vi "Camera.v9.vi"() -> ()   [LabVIEW 2015]
uses:
  Camera Properties.ctl
  Microscope Settings.ctl
  CameraState.ctl
  ModeEnum.ctl
  Stack_State.ctl
  Stack Track.ctl
  CameraControlTypeDef.ctl
  <vilib>/DAQmx/write.llb/DAQmx Write (Digital 1D Wfm NChan NSamp).vi
  <vilib>/DAQmx/write.llb/DAQmx Write (Analog 1D Wfm NChan NSamp).vi
  <vilib>/DAQmx/create/channels.llb/DAQmx Create Channel (DO-Digital Output).vi
  <vilib>/DAQmx/create/channels.llb/DAQmx Create Channel (AO-Voltage-Basic).vi
  <vilib>/Waveform/WDTOps.llb/WDT Number of Waveform Samples DBL.vi
  <vilib>/DAQmx/configure/timing.llb/DAQmx Timing (Sample Clock).vi
  <vilib>/Waveform/DWDTOps.llb/DWDT Uncompress Digital.vi
  <vilib>/DAQmx/miscellaneous.llb/DAQmx Fill In Error Info.vi
  <vilib>/vision/NI_Vision_Development_Module.lvlib
panel:
  in  "Tab Control":enum32{"Camera Settings", "Recording"}(tab)
  in  "Microscope Settings Array":T1[](array[typedef]) {"Colour 2"."Filter" items=["Empty"=1, ""=2, ""=3, "561"=4, ""=5, "488"=6]; "Z Axis Stepping"."End" min=0.0 max=10.0 step=0.05; "Z Axis Stepping"."Step" min=0.0 max=10.0 step=0.05; "Z Axis Stepping"."Start" min=0.0 max=10.0 step=0.05; "ROI"."y" min=0.0 max=10.0 step=0.05; "ROI"."x" min=0.0 max=10.0 step=0.05; "ROI"."Width" min=0.0 max=10.0 step=0.05; "ROI"."Height" min=0.0 max=10.0 step=0.05; "Camera Delay" min=0.0 max=10.0 step=0.05; "Trigger Source" items=["Internal"=1.0, "External"=2.0]; "Readout Direction" items=["Internal"=1.0, "External"=2.0]; "Slit"."Scanning Mode" items=["Full Frame"=1.0, "Slit Scanning"=12.0]; "Piezo Position /um" min=0.0 max=10.0 step=0.05; "Relax/ms" min=0.0 max=10.0 step=0.05}
  in  "Scan":bool
  in  "Scan Continuously":bool
  out "error IO":errorcluster
  in  "Advanced DCAM Controls":i32(listbox) caption="Multicolumn Listbox"
  in  "Properties":T2=4211904 items=["SENSOR MODE"=4212128, "CCD MODE"=4212384, "READOUT MODE"=4211872, "ACTIVE VIEW INDEX"=4343136, "BITS PER CHANNEL"=4342976, "IMAGE PIXEL TYPE"=4343296, "BINNING"=4215968, "EXPOSURE TIME"=2049184, "CONTRAST GAIN"=3163312, "CONTRAST OFFSET"=3163328, "LIGHT MODE"=2114720, "SENSITIVITY"=2114992, "PHOTON IMAGING MODE"=2115200, "HIGH DYNAMIC RANGE MODE"=3163360, "WHITE BALANCE"=3163568, "TEMPERATURE"=2115232, "TEMPERATURE TARGET"=2115264, "SENSOR COOLER FAN"=2115296, "LINEBUNDLE HEIGHT"=4212192, "MECHANICAL SHUTTER"=2115488, "BACK FOCUS POSITION"=8422304, "TRIGGER CONNECTOR"=1066432, "TRIGGER SOURCE"=1066144, "OUTPUT TRIGGER SOURCE"=1852576, "TRIGGER GLOBAL EXPOSURE"=2049680, "FIRST TRIGGER BEHAVIOR"=2049696, "CHANNEL SYNC"=1852352, "READOUT DIRECTION"=4211904, "PRE HSYNC COUNT"=1852704, "INTERNAL LINE SPEED"=4191408, "INTERNAL LINE INVERVAL"=4191424]
  out "Image":T3(plugin-control)
  out "Histogram":T4(graph)
  in  "stop":bool
  in  "Signals Debugger":bool
  in  "Calibration":bool
  in  "MultiD Scan":bool
  in  "Stage Controller":bool
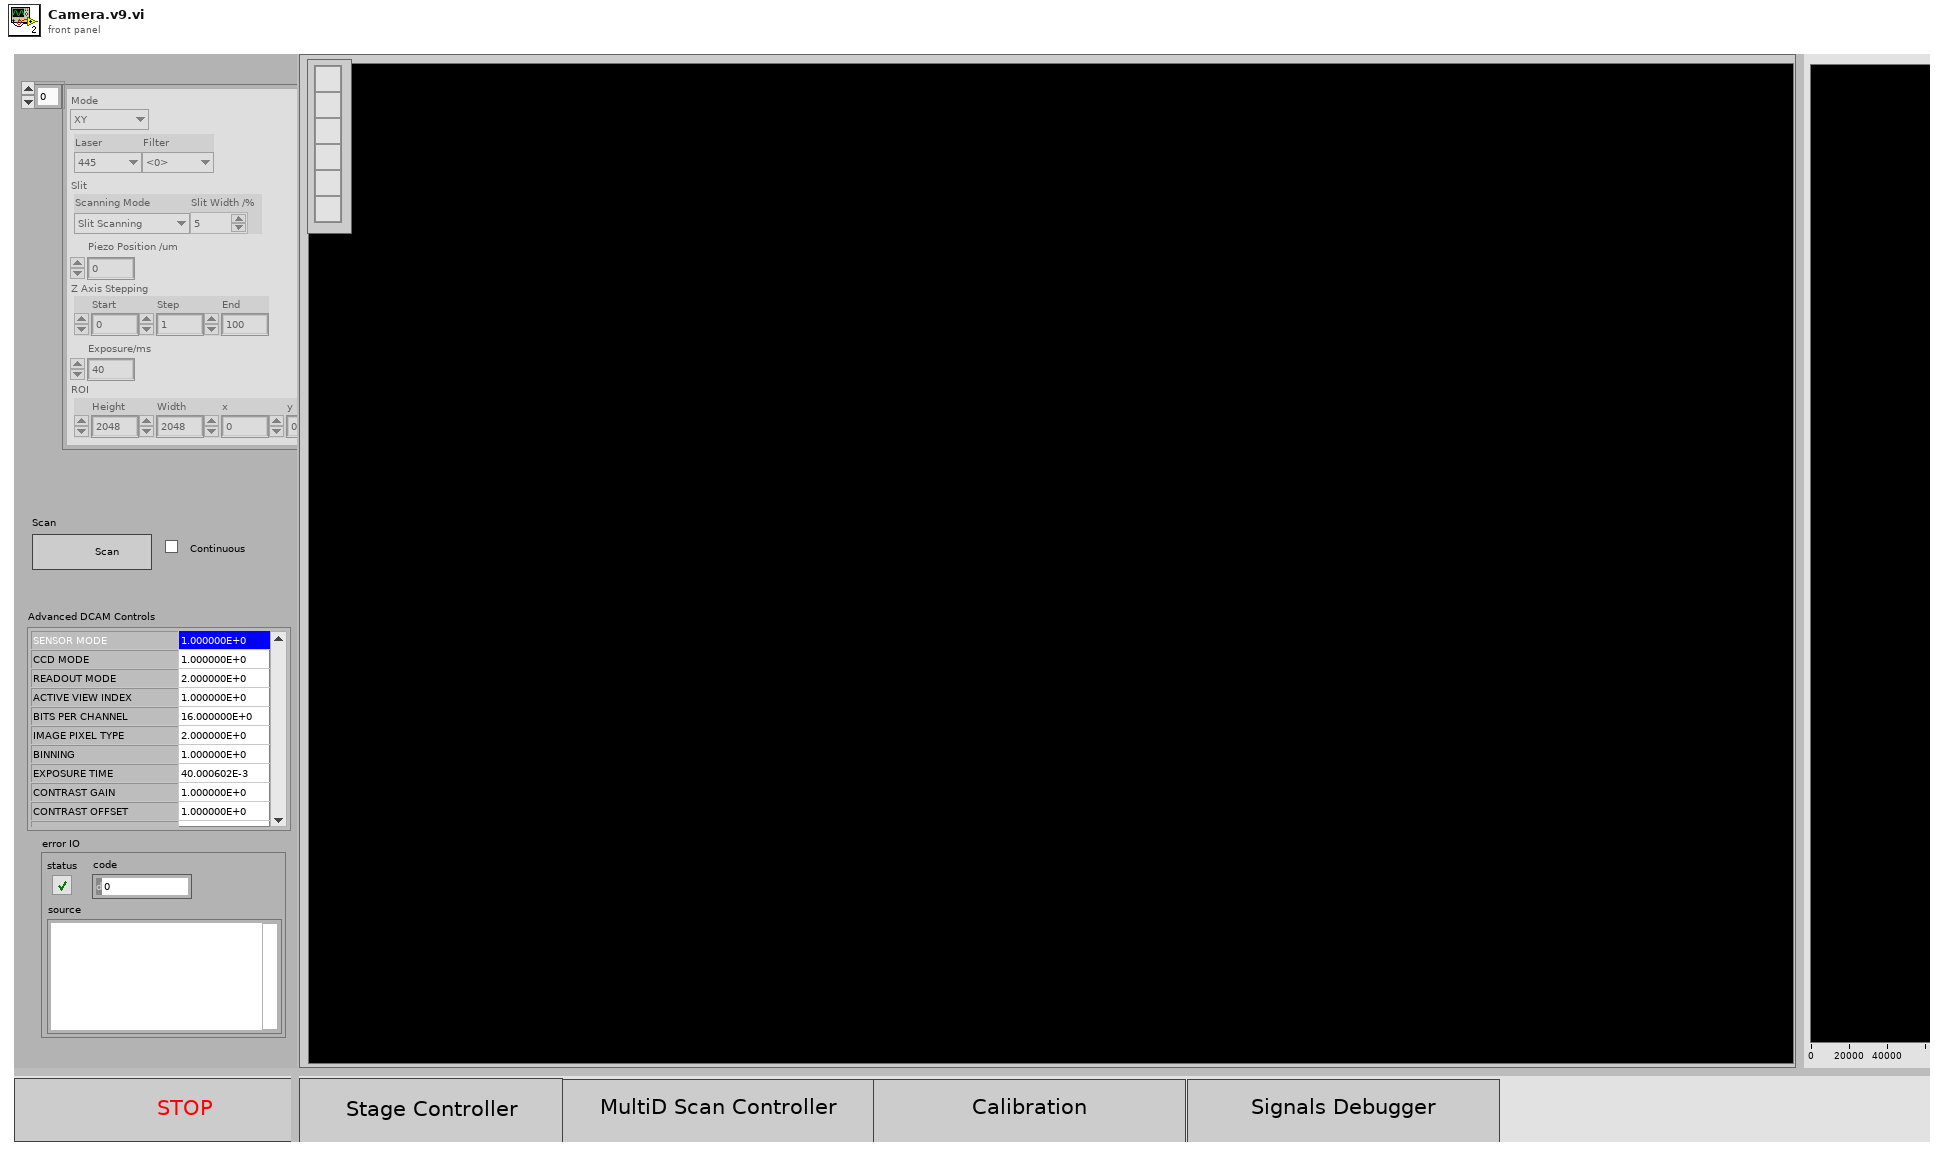
[diagram p1: front panel]
types:
  T1 = typedef "Microscope Settings.ctl" = cluster{"Mode":enum16{"X", "XY", "XYZ", "XYZT", "XYZC"}, "Colour 2":cluster{"Laser":enum16{"445", "488", "561", "647"}, "Filter":u16}, "Slit":cluster{"Scanning Mode":dbl, "Slit Width /%":dbl}, "Piezo Position /um":dbl, "Z Axis Stepping":cluster{"Start":dbl, "Step":dbl, "End":dbl}, "Exposure/ms":dbl, "ROI":cluster{"Height":dbl, "Width":dbl, "x":dbl, "y":dbl}, "Samples per millisecond":dbl, "Relax/ms":dbl, "Readout Direction":dbl, "Trigger Source":dbl, "Camera Delay":dbl}
  T2 = typedef "Camera Properties.ctl" = u32
  T3 = typedef "IMAQ Image.ctl" = refnum<image>
  T4 = cluster{"Starting Value":sgl, "Incremental Value":sgl, "Histogram":u32[]}
  T5 = cluster{"height":u32, "width":u32, "datatype":u32}
  T6 = typedef "CameraState.ctl" = enum16{"init", "active", "deinit"}
  T7 = typedef "ModeEnum.ctl" = enum16{"Idle", "generateWaves", "runWaves", "stop"}
  T8 = typedef "CameraControlTypeDef.ctl" = enum16{"Idle", "IntervalLineInt", "Ram Record", "HardDisk Record", "Disengage Update", "Update", "ROI", "Binning", "Scan Mode", "Trigger Mode", "Readout Mode", "Readout Direction", "Preview", "ROIWindow", "Trigger Source"}
  T9 = cluster{"Mode":u32, "Polarity":u32, "Times":u32, "Delay":dbl}
  T10 = typedef "Stack_State.ctl" = cluster{"State":T11, "Stack Number":i32, "Image":u16[][], "Stacks":i32}
  T11 = typedef "Stack Track.ctl" = enum16{"Idle", "Display", "Start Sequence", "Read Disk", "STOP", "Collecting", "End"}
  T12 = enum32{"Invalid", "Standard", "Closed", "Hidden", "Minimized", "Maximized"}
  T13 = typedef "Image Type" = u32
  T14 = cluster{"Enum":T8, "Microscope Settings Array":T1[]}
  T15 = cluster{"Mode":T7, "Microscope Settings Array":T1[]}
  T16 = cluster{"State":T11, "Timeout":i32, "Data 16":u16[][], "Timeout":i32}
  T17 = cluster{waveform(dbl)[], "Digital Waveform":digitalwaveform, "Digital Waveform":digitalwaveform}
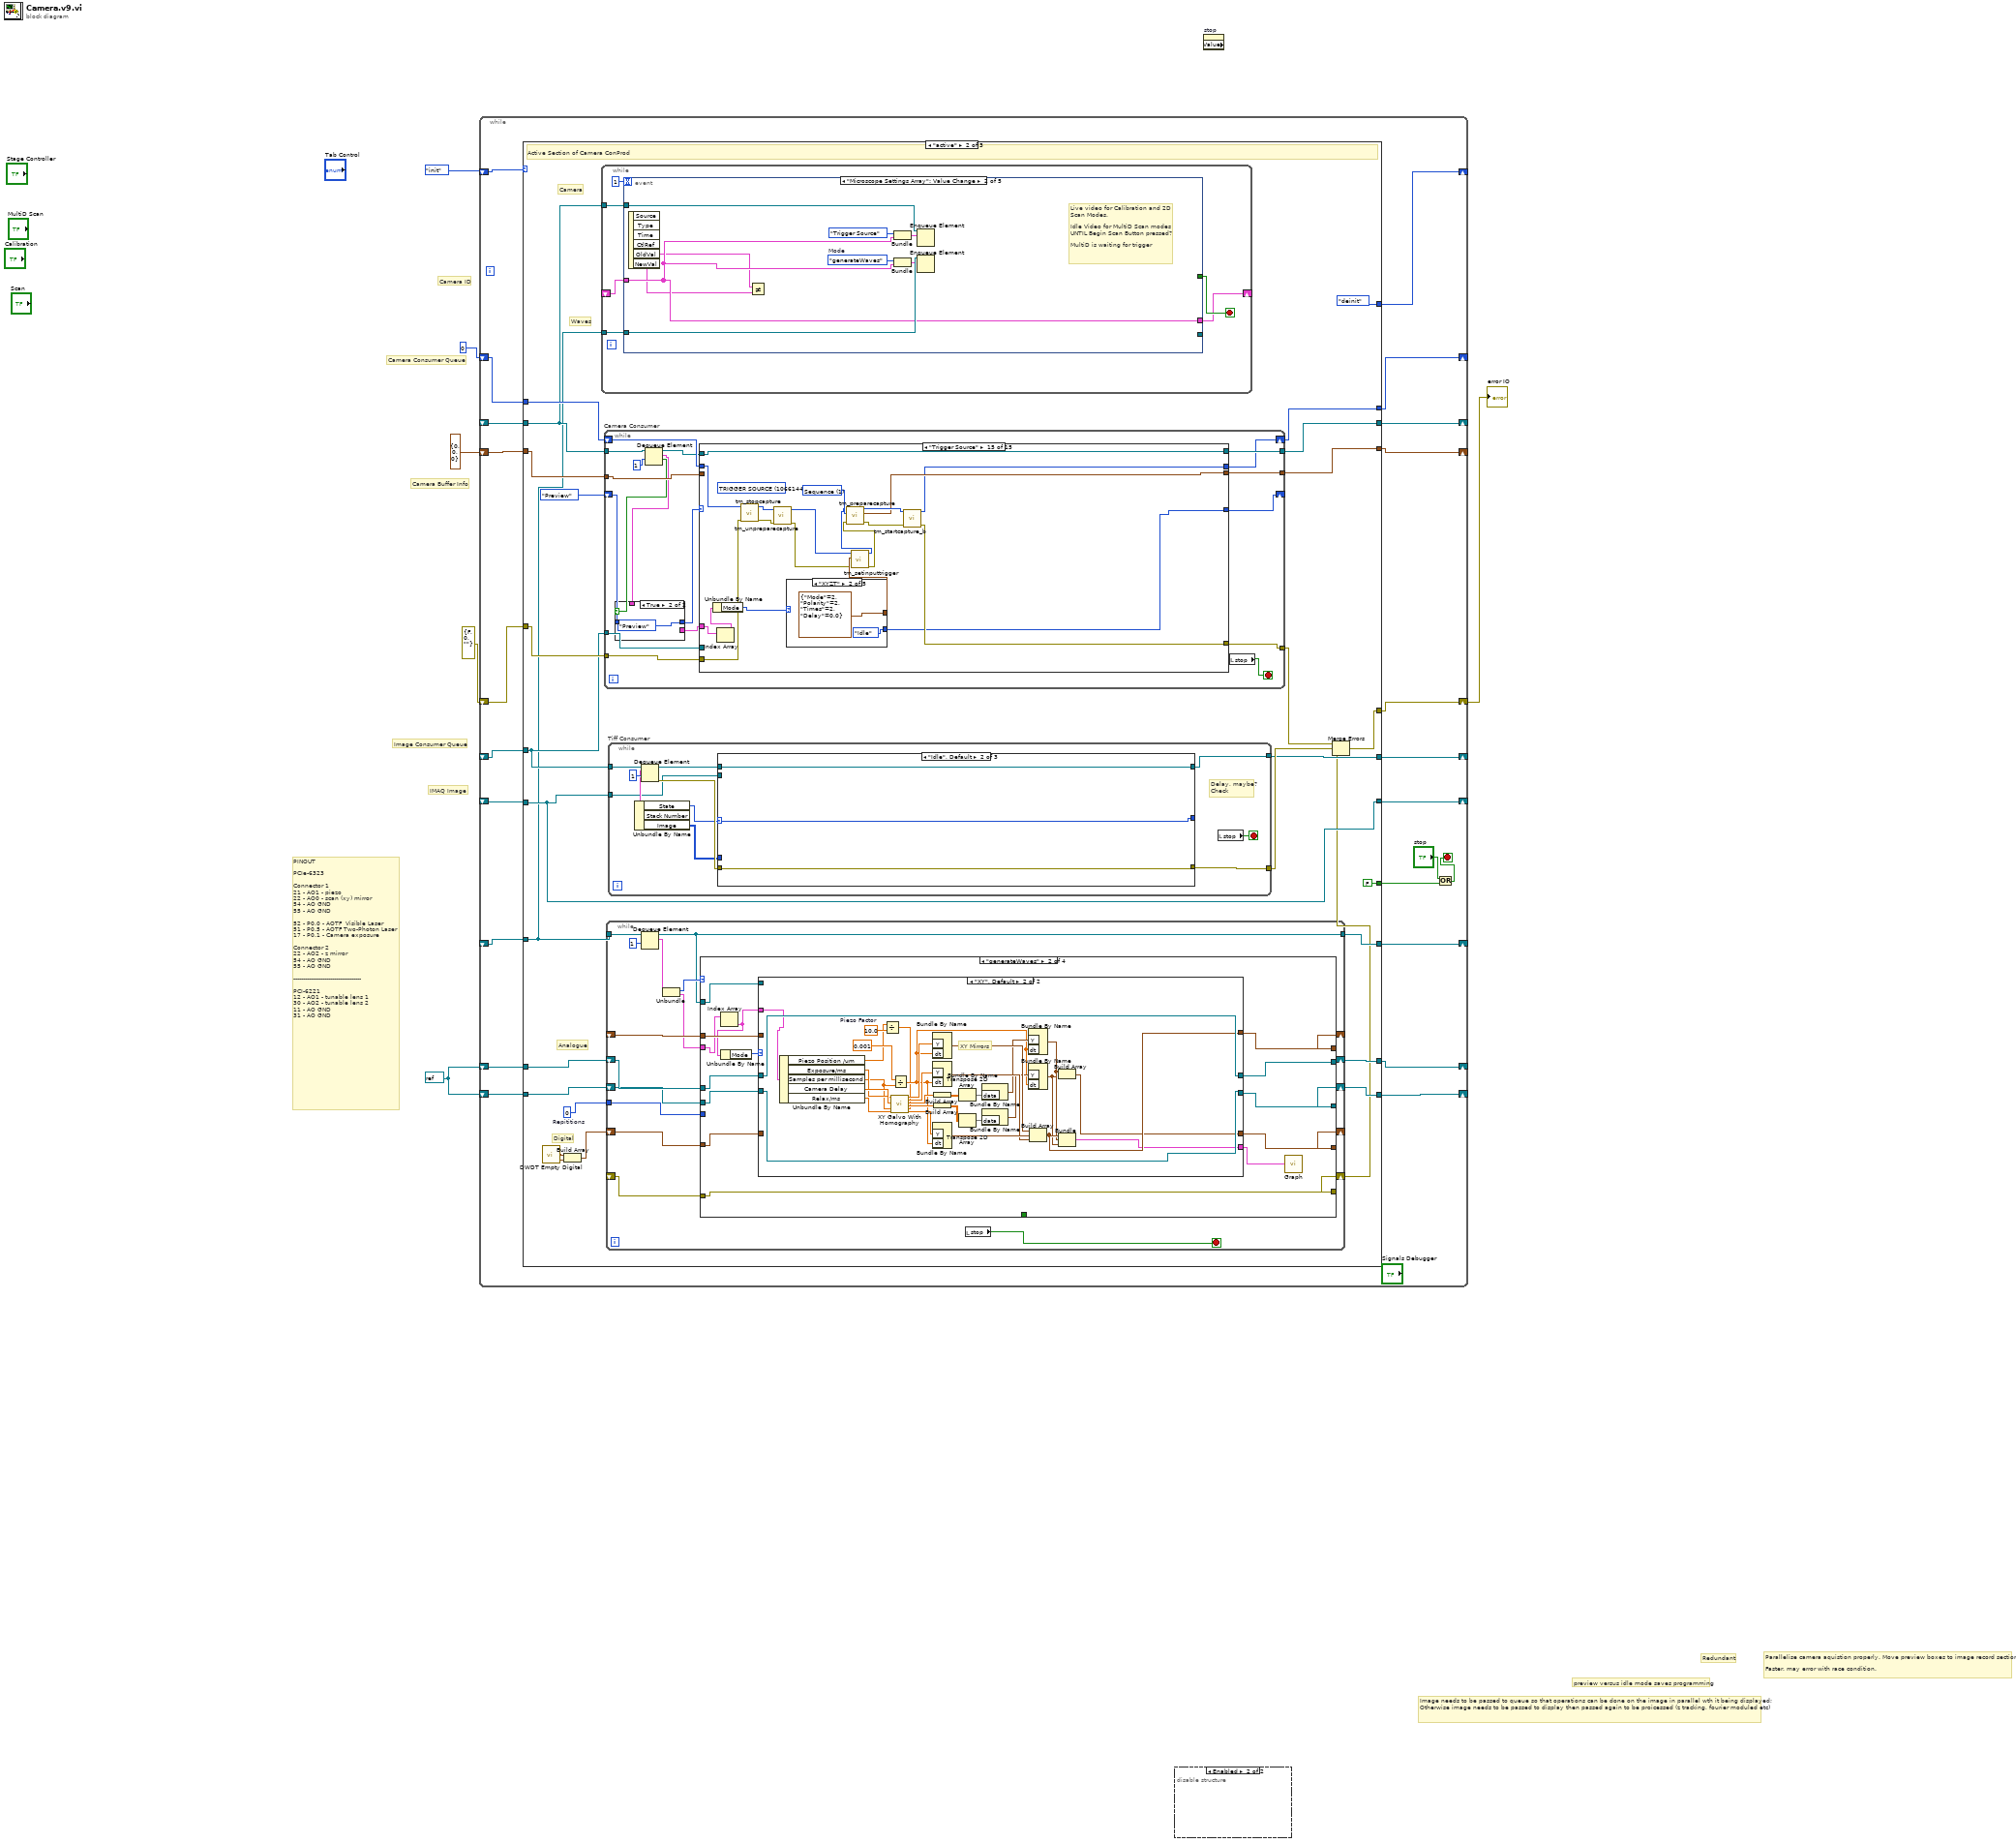
[diagram p0: block diagram]
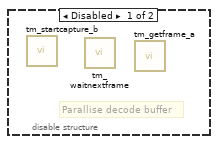
[diagram p2: hidden frame]
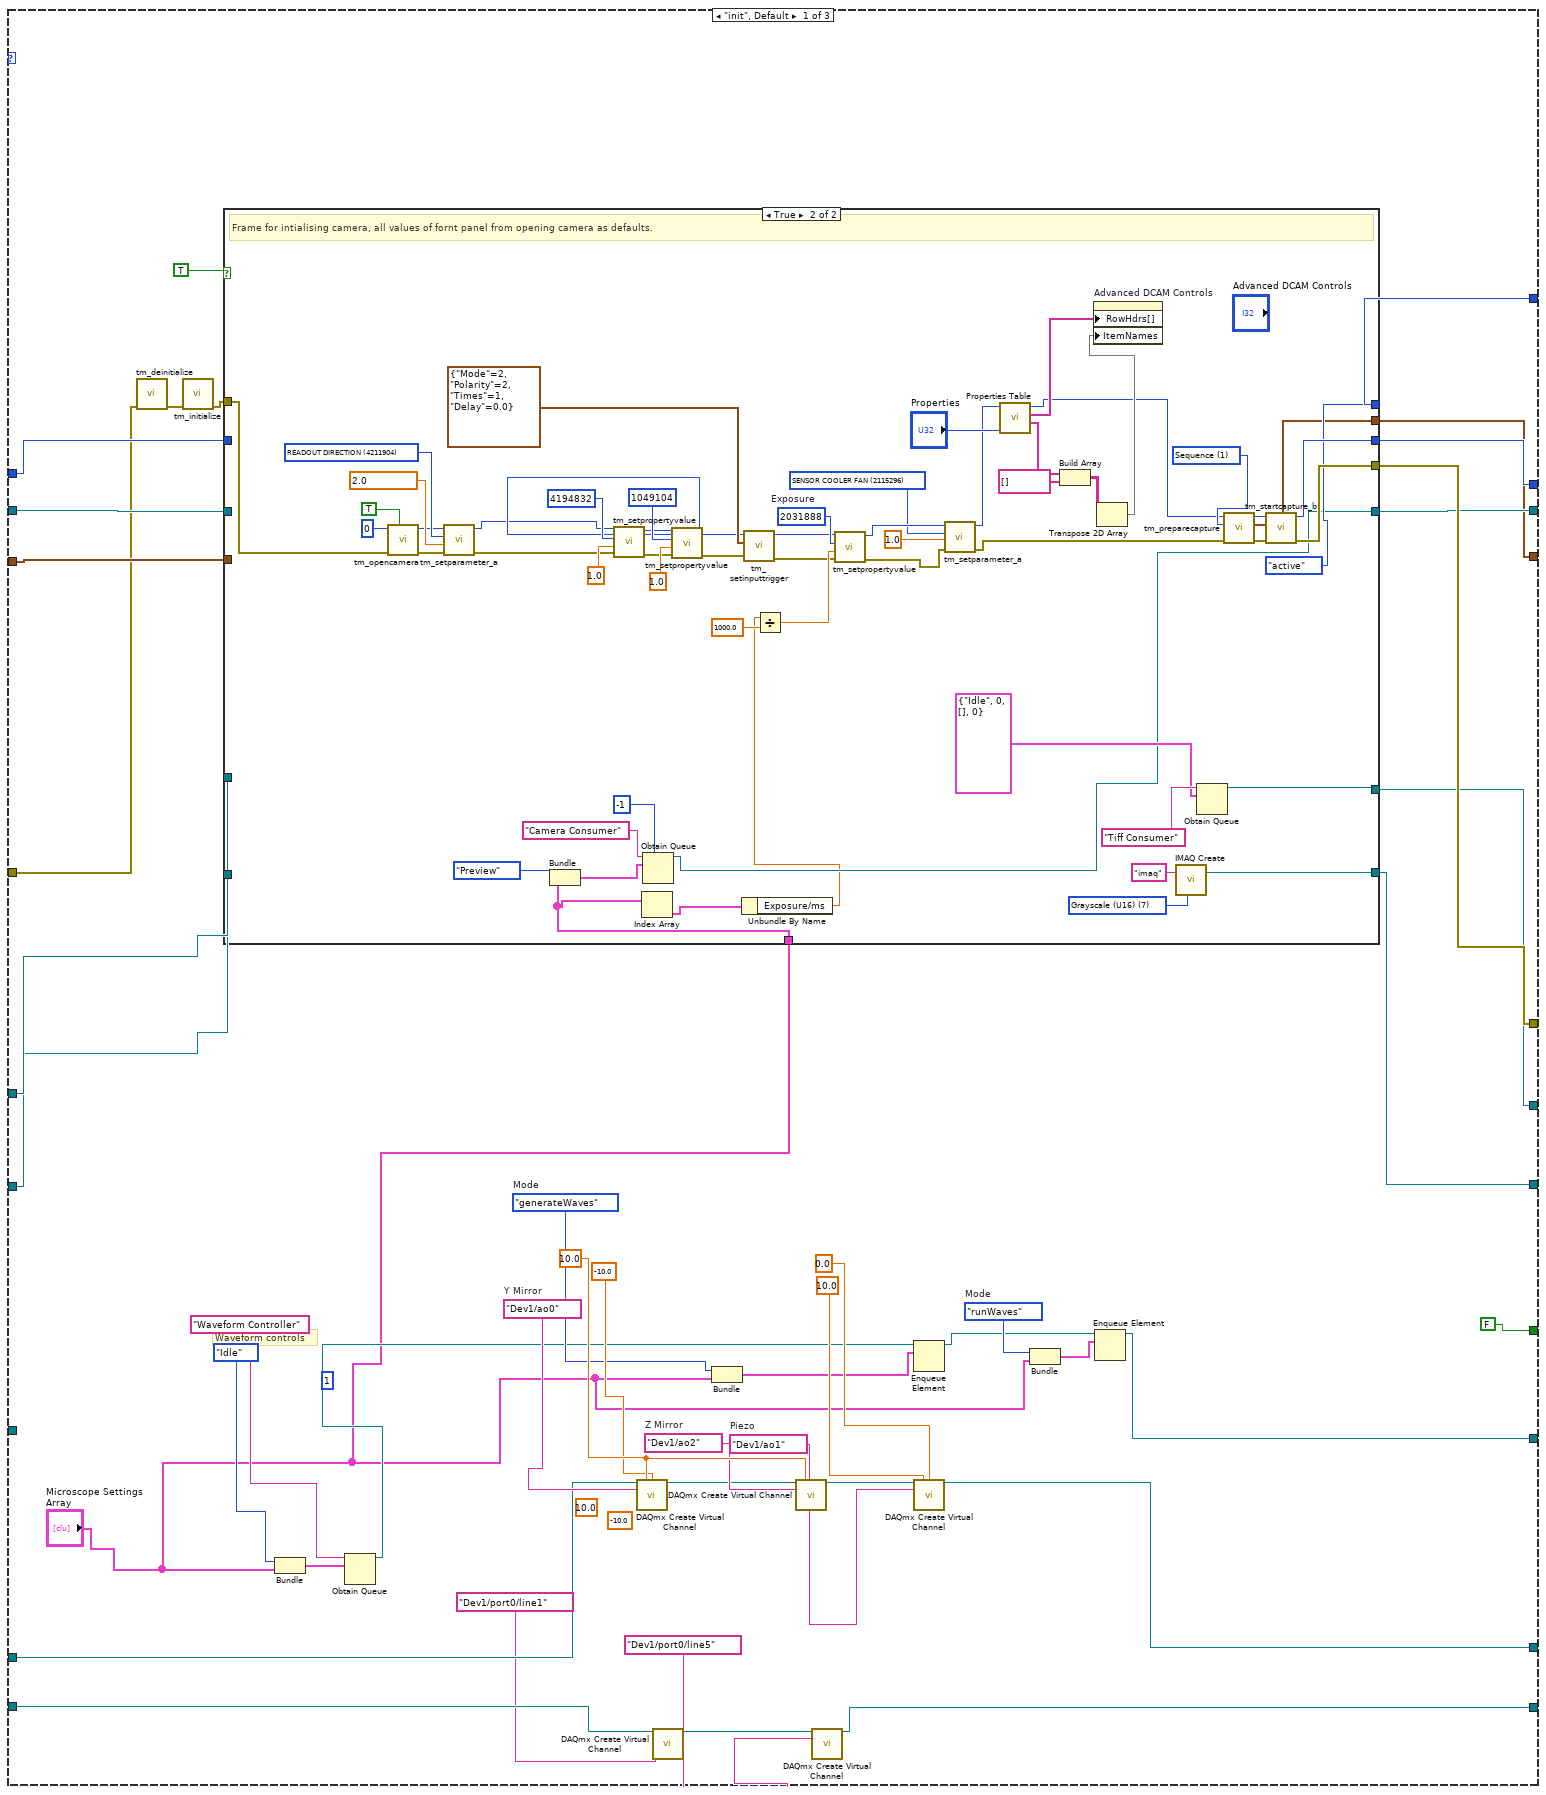
[diagram p3: hidden frame]
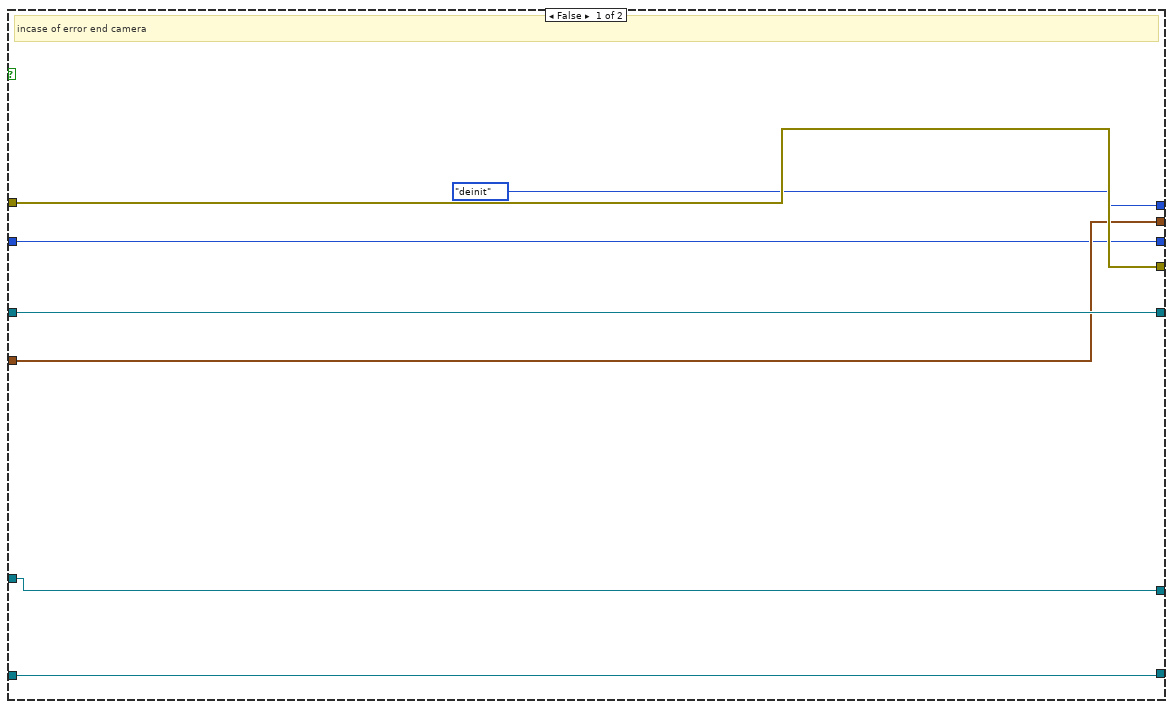
[diagram p4: hidden frame]
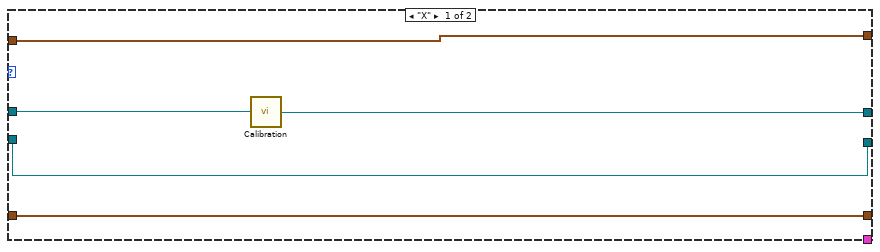
[diagram p6: hidden frame]
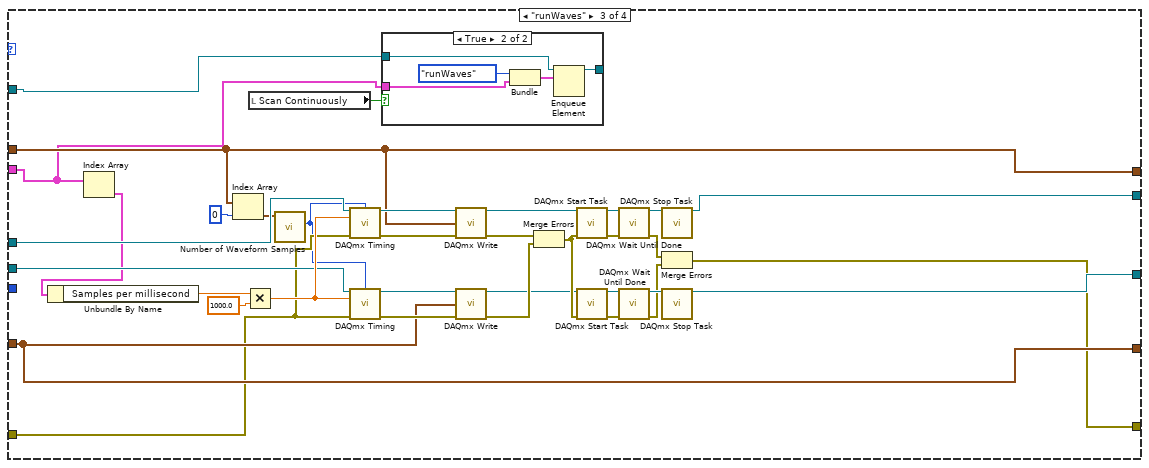
[diagram p7: hidden frame]
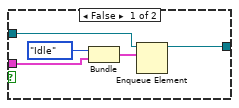
[diagram p8: hidden frame]
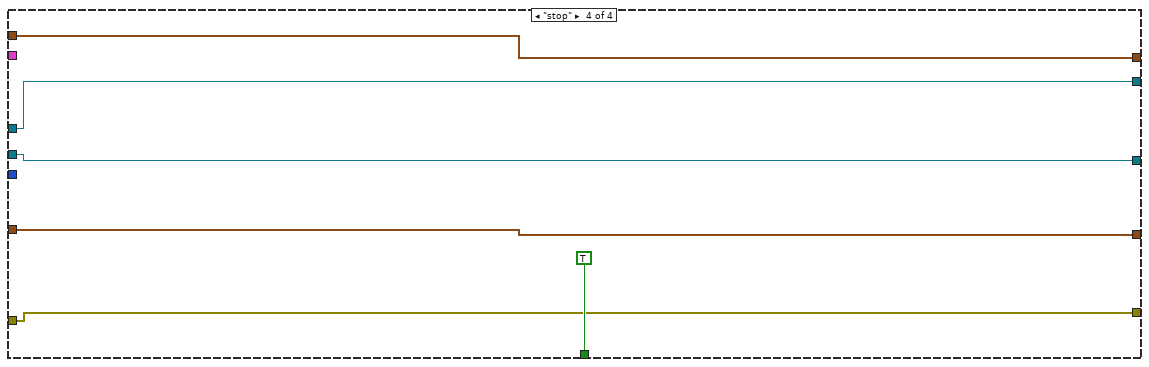
[diagram p9: hidden frame]
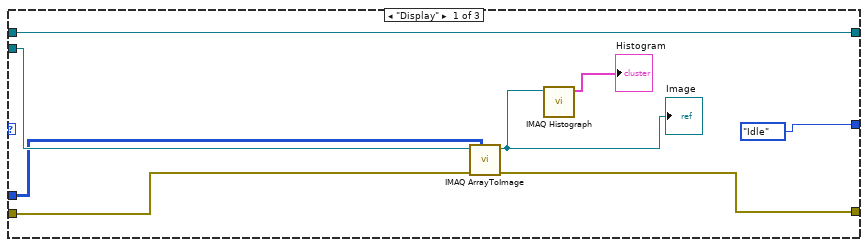
[diagram p10: hidden frame]
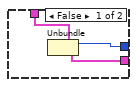
[diagram p12: hidden frame]
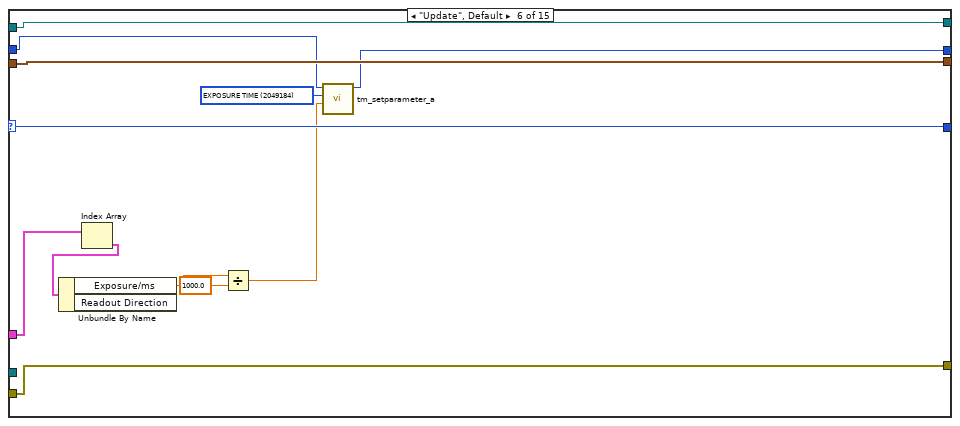
[diagram p18: hidden frame]
diagram:
  w3 = refnum<k21> refnum ("Mirror Z 2")
  # "PINOUT\n\nPCIe-6323\n\nConnector 1\n21 - AO1 - piezo\n22 - AO0 - scan (xy) mirror\n54 - AO GND\n55 - AO GND\n\n52 - P0.0 - AOTF  Visible Laser\n51 - P0.5 - AOTF Two-Photon Laser\n17 - P0.1 - Camera exposure\n\nConnector 2\n22 - AO2 - z mirror\n54 - AO GND\n55 - AO GND\n\n-----------------------------------\n\nPCI-6221\n12 - AO1 - tunable lens 1\n30 - AO2 - tunable lens 2\n11 - AO GND\n31 - AO GND"
  # "IMAQ Image"
  # "Camera Buffer Info"
  # "Image needs to be passed to queue so that operations can be done on the image in parallel wth it being displayed;\nOtherwise image needs to be passed to display then passed again to be proicessed (z tracking, fourier moduled etc)"
  # "preview versus idle mode saves programming"
  # "Parallelise camera aquistion properly. Move preview boxes to image record section.\n\nFaster. may error with race condition."
  # "Redundant"
  # "Image Consumer Queue"
  # "Camera Consumer Queue"
  # "Camera ID"
  n1 = while {
    shift-right: [w29] -> _
    shift-left: CameraState."init" -> [w28]
    shift-right: [w27] -> _
    shift-left: u32 0 ("Handle out") -> [w26]
    shift-right: [w25] -> w5
    shift-left: errorcluster {"status"=FALSE, "code"=0, "source"=""} ("error IO") -> [w24]
    shift-right: [w22] -> _
    shift-left: _ -> [w21]
    shift-right: [w23] -> _
    shift-left: _ -> [w20]
    shift-right: [w16] -> _
    shift-left: T5 {"height"=0, "width"=0, "datatype"=0} ("Buffer Info") -> [w15]
    shift-right: [w14] -> _
    shift-left: _ -> [w13]
    shift-right: [w12] -> _
    shift-left: w3 -> [w11]
    shift-right: [w9] -> _
    shift-left: w3 -> [w10]
    shift-right: [w8] -> _
    shift-left: _ -> [w7]
    stop <- w18 stop-if-true
    n2 = case shown="\"active\"" w28 {
      tunnel: [w71 CameraState."deinit" CameraState."init"] -> w29
      tunnel: [w70 w162 w555] -> w27
      tunnel: w26 -> [w48 w163 w555]
      tunnel: [w69 w161 w558] -> w25
      tunnel: w24 -> [w47 w155 w559]
      tunnel: [w68 w158 w542] -> w23
      tunnel: [w67 w157 w538] -> w22
      tunnel: w21 -> [w65 w150 w538]
      tunnel: w20 -> [w66 w148 w542]
      tunnel: [FALSE ("stop") FALSE ("stop") TRUE ("stop")] -> w17
      tunnel: [w63 w153 w552] -> w16
      tunnel: w15 -> [w62 w152 w552]
      tunnel: w13 -> [w60 w149 w551]
      tunnel: [w61 w149 w551] -> w14
      tunnel: w7 -> [_ w140 w537]
      tunnel: [w52 w141 w549] -> w12
      tunnel: w11 -> [w49 w144 w549]
      tunnel: w10 -> [w45 w143 w547]
      tunnel: [w40 w142 w547] -> w9
      tunnel: [w31 w139 w537] -> w8
      frame "init", Default {
        w35 = ModeEnum."runWaves"  # Mode
        (unwired) 1 ("max queue size (-1, unlimited)")
        w44 = ModeEnum."generateWaves"  # Mode
        (unwired) -10.0 ("minimum value")
        (unwired) 10.0 ("maximum value")
        w55 = tag "Dev1/ao1"  # Piezo
        w56 = tag "Dev1/ao2"  # Z Mirror
        w57 = tag "Dev1/ao0"  # Y Mirror
        w59 = 10.0 ("maximum value")
        # "Waveform controls"
        n3 = call "tm_deinitialize.vi"("error in (no error)"=w47) -> ("error out"=w73:errorcluster)  [unwired: 10 in]
        n4 = call "tm_initialize.vi"("error in (no error)"=w73) -> ("error out"=w72:errorcluster)  [unwired: 7 in, 3 out]
        n5 = case shown="True" TRUE {
          tunnel: w72 -> [w80 w102]
          tunnel: [CameraState."deinit" CameraState."active"] -> w71
          tunnel: [w80 w133] -> w69
          tunnel: [w75 w131] -> w70
          tunnel: [w78 w121] -> w68
          tunnel: [w77 w128] -> w67
          tunnel: w66 -> [w78 _]
          tunnel: w65 -> [w77 _]
          tunnel: [w76 w126] -> w63
          tunnel: w62 -> [w76 _]
          tunnel: w48 -> [w75 _]
          tunnel: [w74 w123] -> w61
          tunnel: w60 -> [w74 _]
          tunnel: "Microscope Settings Array" -> [_ w81]
          frame False {
            # "incase of error end camera"
          }
          frame True {
            w99 = u32 2115296 items=["SENSOR MODE"=4212128, "CCD MODE"=4212384, "READOUT MODE"=4211872, "ACTIVE VIEW INDEX"=4343136, "BITS PER CHANNEL"=4342976, "IMAGE PIXEL TYPE"=4343296, "BINNING"=4215968, "EXPOSURE TIME"=2049184, "CONTRAST GAIN"=3163312, "CONTRAST OFFSET"=3163328, "LIGHT MODE"=2114720, "SENSITIVITY"=2114992, "PHOTON IMAGING MODE"=2115200, "HIGH DYNAMIC RANGE MODE"=3163360, "WHITE BALANCE"=3163568, "TEMPERATURE"=2115232, "TEMPERATURE TARGET"=2115264, "SENSOR COOLER FAN"=2115296, "LINEBUNDLE HEIGHT"=4212192, "MECHANICAL SHUTTER"=2115488, "BACK FOCUS POSITION"=8422304, "TRIGGER CONNECTOR"=1066432, "TRIGGER SOURCE"=1066144, "OUTPUT TRIGGER SOURCE"=1852576, "TRIGGER GLOBAL EXPOSURE"=2049680, "FIRST TRIGGER BEHAVIOR"=2049696, "CHANNEL SYNC"=1852352, "READOUT DIRECTION"=4211904, "PRE HSYNC COUNT"=1852704, "INTERNAL LINE SPEED"=4226000, "INTERNAL LINE INTERVAL"=4226016] ("Parameter")
            w108 = u32 2031888  # Exposure
            w119 = sgl 2.0 items=["Forward"=1.0, "Backward"=2.0] ("Readout Direction")
            w120 = u32 4211904 items=["SENSOR MODE"=4212128, "CCD MODE"=4212384, "READOUT MODE"=4211872, "ACTIVE VIEW INDEX"=4343136, "BITS PER CHANNEL"=4342976, "IMAGE PIXEL TYPE"=4343296, "BINNING"=4215968, "EXPOSURE TIME"=2049184, "CONTRAST GAIN"=3163312, "CONTRAST OFFSET"=3163328, "LIGHT MODE"=2114720, "SENSITIVITY"=2114992, "PHOTON IMAGING MODE"=2115200, "HIGH DYNAMIC RANGE MODE"=3163360, "WHITE BALANCE"=3163568, "TEMPERATURE"=2115232, "TEMPERATURE TARGET"=2115264, "SENSOR COOLER FAN"=2115296, "LINEBUNDLE HEIGHT"=4212192, "MECHANICAL SHUTTER"=2115488, "BACK FOCUS POSITION"=8422304, "TRIGGER CONNECTOR"=1066432, "TRIGGER SOURCE"=1066144, "OUTPUT TRIGGER SOURCE"=1852576, "TRIGGER GLOBAL EXPOSURE"=2049680, "FIRST TRIGGER BEHAVIOR"=2049696, "CHANNEL SYNC"=1852352, "READOUT DIRECTION"=4211904, "PRE HSYNC COUNT"=1852704, "INTERNAL LINE SPEED"=4226000, "INTERNAL LINE INTERVAL"=4226016] ("Parameter")
            w125 = T13 7 items=["Grayscale (U8)", "Grayscale (I16)", "Grayscale (SGL)", "Complex (CSG)", "RGB (U32)", "HSL (U32)", "RGB (U64)", "Grayscale (U16)"] ("Image Type")
            w135 = 1 items=["Snap", "Sequence"] ("Capture mode")
            # "Frame for intialising camera, all values of fornt panel from opening camera as defaults."
            n6 = call "tm_opencamera.vi"("Force Open"=TRUE, "error in (no error)"=w102, "Camera Index"=u32 0) -> ("error out"=w117:errorcluster, "Handle out"=w118:u32)  [unwired: 6 in, 1 out]
            n7 = call "tm_setparameter_a.vi"("error in (no error)"=w117, "Value in"=w119, "Parameter"=w120, "Handle in"=w118) -> ("error out"=w88:errorcluster, "Handle out"=w109:u32)  [unwired: 6 in]
            n8 = Bundle("Enum"=CameraControlTypeDef."Preview", "Microscope Settings Array"=w81) -> (w103:T14)  [unwired: 1 in]
            n9 = call "tm_setpropertyvalue.vi"("error in (no error)"=w88, "Value in"=sgl 1.0, "Property ID"=u32 4194832, "Handle in"=w109) -> ("error out"=w87:errorcluster, "Handle out"=w112:u32)  [unwired: 6 in]
            n10 = Index Array(array=w81) -> (element=w82:T1)  [unwired: 1 in]
            n11 = Obtain Queue(max queue size (-1, unlimited)=-1, name (unnamed)="Camera Consumer", element data type=w103) -> (queue out=w121:refnum<queue>)  [unwired: 2 in, 2 out]
            n12 = call "tm_setpropertyvalue.vi"("error in (no error)"=w87, "Value in"=sgl 1.0, "Property ID"=u32 1049104, "Handle in"=w112) -> ("error out"=w86:errorcluster, "Handle out"=w110:u32)  [unwired: 6 in]
            n13 = Unbundle By Name(w82) -> ("Exposure/ms"=w89:dbl)
            n14 = call <userlib>:"tm_setinputtrigger.vi"("error in (no error)"=w86, "Parameters"=T9 {"Mode"=2, "Polarity"=2, "Times"=1, "Delay"=0.0}, "Handle in"=w110) -> ("error out"=w85:errorcluster, "Handle out"=w107:u32)  [unwired: 7 in]
            n15 = Divide(x=w89, y=sgl 1000.0) -> (x/y=w105:dbl)
            n16 = call "tm_setpropertyvalue.vi"("error in (no error)"=w85, "Value in"=w105, "Property ID"=w108, "Handle in"=w107) -> ("error out"=w84:errorcluster, "Handle out"=w100:u32)  [unwired: 6 in]
            n17 = call "tm_setparameter_a.vi"("error in (no error)"=w84, "Value in"=1.0, "Parameter"=w99, "Handle in"=w100) -> ("error out"=w83:errorcluster, "Handle out"=w91:u32)  [unwired: 6 in]
            n18 = call "Properties Table.vi"("Properties"="Properties", "Handle In"=w91) -> ("Value Stirngs Out"=w95:string[], "Row Headers"=w96:string[], "Handle Out"=w90:u32)  [unwired: 3 in, 1 out]
            n19 = Build Array(w95, string[] [] ("element")) -> (w93:string[][])
            n20 = Transpose 2D Array(2D array=w93) -> (transposed array=w92:string[][])
            n21 = property on="Advanced DCAM Controls" class="MCListbox (strict)"("RowHdrs[]"=w96, "ItemNames"=w92) -> ()  [unwired: 2 in, 2 out]
            n22 = call "IMAQ Create"("Image Name"="imaq", "Image Type"=w125) -> ("New Image"=w123:T3)  [unwired: 3 in, 1 out]
            n23 = Obtain Queue(name (unnamed)="Tiff Consumer", element data type=T10 {"State"=enum."Idle", "Stack Number"=0, "Image"=[], "Stacks"=0} ("input cluster")) -> (queue out=w128:refnum<queue>)  [unwired: 3 in, 2 out]
            n24 = call "tm_preparecapture.vi"("error in (no error)"=w83, "Capture mode"=w135, "Handle in"=w90) -> ("error out"=w134:errorcluster, "Buffer Info"=w126:T5, "Handle out"=w132:u32)  [unwired: 5 in, 1 out]
            n25 = call "tm_startcapture_b.vi"("error in (no error)"=w134, "Handle in"=w132) -> ("error out"=w133:errorcluster, "Handle out"=w131:u32)  [unwired: 8 in]
          }
        }
        n26 = Bundle("Mode"=ModeEnum."Idle", "Microscope Settings Array"="Microscope Settings Array") -> (w42:T15)  [unwired: 1 in]
        n27 = Obtain Queue(name (unnamed)="Waveform Controller", element data type=w42) -> (queue out=w41:refnum<queue>)  [unwired: 3 in, 2 out]
        n28 = call-poly <vilib>:"DAQmx Create Virtual Channel.vi"("task in"=w49, "maximum value"=w59, "minimum value"=-10.0, "physical channels"=w57) -> ("task out"=w51:refnum<k21>)  [unwired: 10 in, 1 out]
        n29 = call-poly <vilib>:"DAQmx Create Virtual Channel.vi"("task in"=w45, "lines"=tag "Dev1/port0/line1") -> ("task out"=w46:refnum<k21>)  [unwired: 12 in, 1 out]
        n30 = Bundle("Mode"=w44, "Microscope Settings Array"="Microscope Settings Array") -> (w33:T15)  [unwired: 1 in]
        n31 = call-poly <vilib>:"DAQmx Create Virtual Channel.vi"("task in"=w51, "maximum value"=w59, "physical channels"=w56) -> ("task out"=w50:refnum<k21>)  [unwired: 11 in, 1 out]
        n32 = call-poly <vilib>:"DAQmx Create Virtual Channel.vi"("task in"=w46, "lines"=tag "Dev1/port0/line5") -> ("task out"=w40:refnum<k21>)  [unwired: 12 in, 1 out]
        n33 = Enqueue Element(queue=w41, element=w33) -> (queue out=w34:refnum<queue>)  [unwired: 2 in, 2 out]
        n34 = call-poly <vilib>:"DAQmx Create Virtual Channel.vi"("task in"=w50, "maximum value"=10.0 ("minimum value"), "minimum value"=0.0 ("maximum value"), "physical channels"=w55) -> ("task out"=w52:refnum<k21>)  [unwired: 10 in, 1 out]
        n35 = Bundle("Mode"=w35, "Microscope Settings Array"="Microscope Settings Array") -> (w32:T15)  [unwired: 1 in]
        n36 = Enqueue Element(queue=w34, element=w32) -> (queue out=w31:refnum<queue>)  [unwired: 2 in, 2 out]
      }
      frame "active" {
        w147 = 0  # Repititions
        # "Waves"
        # "Camera"
        # "Digital"
        # "Analogue"
        # "Active Section of Camera ConProd"
        n37 = call <vilib>:"DWDT Empty Digital.vi"() -> ("digital waveform out"=w145:digitalwaveform)  [unwired: 5 in]
        n38 = Build Array(w145, w145) -> (w146:digitalwaveform[])
        n39 = while {
          tunnel: w148 -> [w503]
          shift-right: [w502] -> _
          shift-left: _ -> [w501]
          tunnel: w140 -> [w499]
          stop <- w504 stop-if-true
          n40 = event shown="[1] \"Microscope Settings Array\": Value Change" {
            selector: _ -> [_ _ _ _ _]
            dyn-events: _ -> [_ _ _ _ _]
            timeout: 1 -> [_ _ _ _ _]
            tunnel: [w512 _ _ _ _] -> w504
            tunnel: w503 -> [w507 w521 _ _ _]
            tunnel: [w505 w515 _ _ w536] -> w502
            tunnel: w501 -> [w505 w515 _ w529 _]
            tunnel: [_ _ _ w528 _] -> _
            tunnel: w499 -> [w506 w520 _ w527 _]
            event "stop": Value Change {
              w510 = ModeEnum."stop"  # Mode
              n41 = event-data() -> ()  [unwired: 1 in, 6 out]
              n42 = Bundle("Enum"=CameraControlTypeDef."Idle", "Value"=w505) -> (w508:cluster{"Enum":T8, "Value":T1[]})  [unwired: 1 in]
              n43 = Bundle("Mode"=w510, "Value"=w505) -> (w509:cluster{"Mode":T7, "Value":T1[]})  [unwired: 1 in]
              n44 = Enqueue Element(queue=w507, element=w508) -> ()  [unwired: 2 in, 3 out]
              n45 = Enqueue Element(queue=w506, element=w509) -> ()  [unwired: 2 in, 3 out]
              n46 = local read "stop"() -> (w512:bool)
            }
            event "Microscope Settings Array": Value Change {
              w518 = ModeEnum."generateWaves"  # Mode
              # "Live video for Calibration and 2D\nScan Modes.\n\nIdle Video for MultiD Scan modes\nUNTIL Begin Scan Button pressed?\n\nMultiD is waiting for trigger"
              n47 = event-data() -> ("OldVal"=w514:T1[], "NewVal"=w513:T1[])  [unwired: 1 in, 4 out]
              n48 = Not Equal?(x=w514, y=w513) -> ()  [unwired: 1 out]
              n49 = Bundle("Enum"=CameraControlTypeDef."Trigger Source", "Value"=w515) -> (w516:cluster{"Enum":T8, "Value":T1[]})  [unwired: 1 in]
              n50 = Bundle("Mode"=w518, "Value"=w515) -> (w517:cluster{"Mode":T7, "Value":T1[]})  [unwired: 1 in]
              n51 = Enqueue Element(queue=w521, element=w516) -> ()  [unwired: 2 in, 3 out]
              n52 = Enqueue Element(queue=w520, element=w517) -> ()  [unwired: 2 in, 3 out]
            }
            event "Signals Debugger": Value Change {
              n53 = event-data() -> ()  [unwired: 1 in, 6 out]
              n54 = disable-structure shown="Disabled" {
                frame Disabled {
                  n55 = control-ref of="stop"() -> (w525:refnum<vi>)
                  n56 = call "PopOutGraph.vi"("OK Button 2"=w525) -> ()  [unwired: 2 in]
                }
                frame Enabled {
                }
              }
              n57 = vi-ref "Graph.vi"() -> (w522:refnum<vi>)
              n58 = invoke class="VI" method="FP.Open"(reference=w522, "Activate"=TRUE ("Front Panel Window:Open"), "State"=T12."Standard") -> ()  [unwired: 2 in, 5 out]
            }
            event "Scan": Value Change {
              n59 = event-data() -> ("NewVal"=w526:bool)  [unwired: 1 in, 5 out]
              n60 = case shown="True" w526 {
                tunnel: w529 -> [_ w535]
                tunnel: [w530 w534] -> w528
                tunnel: w527 -> [w530 w533]
                frame False {
                }
                frame True {
                  w532 = ModeEnum."runWaves"  # Mode
                  n61 = Bundle("Mode"=w532, "Value"=w535) -> (w531:cluster{"Mode":T7, "Value":T1[]})  [unwired: 1 in]
                  n62 = Enqueue Element(queue=w533, element=w531) -> (queue out=w534:refnum<queue>)  [unwired: 2 in, 2 out]
                }
              }
            }
            event Timeout {
              n63 = event-data() -> ()  [unwired: 1 in, 3 out]
              n64 = property on="Microscope Settings Array" class="Arr (strict)"() -> ("Value"=w536:T1[])  [unwired: 2 in, 2 out]
            }
          }
        }
        n65 = while "Camera Consumer" {
          tunnel: w155 -> [w329]
          tunnel: [w314] -> w159
          tunnel: w148 -> [w322]
          tunnel: [w330] -> w158
          shift-right: [w328] -> _
          shift-left: CameraControlTypeDef."Preview" ("Enum") -> [w318]
          tunnel: [w325] -> w153
          tunnel: w152 -> [w324]
          tunnel: w150 -> [w317]
          shift-right: [w326] -> w162
          shift-left: w163 -> [w327]
          stop <- w313 stop-if-true
          n66 = Dequeue Element(queue=w322, timeout in ms (-1)=1) -> (queue out=w321:refnum<queue>, element=w316:T14, timed out?=w320:bool)  [unwired: 1 in, 1 out]
          n67 = case shown="True" w320 {
            tunnel: [w332 CameraControlTypeDef."Preview" ("Enum")] -> w319
            tunnel: w318 -> [_ _]
            tunnel: w316 -> [w333 _]
            tunnel: [w331 _] -> w315
            frame False {
              n68 = Unbundle(w333) -> ("Enum"=w332:T8, "Microscope Settings Array"=w331:T1[])
            }
            frame True {
            }
          }
          n69 = case shown="\"Trigger Source\"" w319 {
            selector: w319 -> [w338 w343 w348 w353 w358 w370 w375 w380 w385 w390 w419 w437 _ w466 _]
            tunnel: w321 -> [w337 w344 w349 w354 w359 w371 w376 w381 w386 w391 _ w433 w448 w468 w488]
            tunnel: [w337 w344 w349 w354 w359 w371 w376 w381 w386 w391 _ w433 w448 w468 w488] -> w330
            tunnel: w329 -> [w339 w342 w347 w352 w357 w369 w374 w379 w384 w389 w414 w436 w440 w465 w479]
            tunnel: [w339 w342 w347 w352 w357 w369 w374 w379 w384 w389 w401 w436 w439 w465 w480] -> w314
            tunnel: [w338 w343 w348 w353 w358 w370 w375 w380 w385 w390 w419 w437 CameraControlTypeDef."Preview" ("Enum") w466 w471] -> w328
            tunnel: w327 -> [w336 w341 w346 w351 w355 w367 w373 w378 w383 w388 w416 w435 w446 w467 w482]
            tunnel: [w336 w341 w346 w351 w355 w366 w373 w378 w383 w388 w394 w435 w444 w467 w481] -> w326
            tunnel: [w335 w340 w345 w350 w356 w368 w372 w377 w382 w387 w418 w434 w442 w464 w483] -> w325
            tunnel: w324 -> [w335 w340 w345 w350 w356 w368 w372 w377 w382 w387 w418 w434 w442 w464 _]
            tunnel: w317 -> [_ _ _ _ _ _ _ _ _ _ _ _ w441 _ _]
            tunnel: w315 -> [_ _ _ _ _ w361 _ _ _ _ w393 _ _ _ w470]
            frame "Idle" {
            }
            frame "IntervalLineInt" {
            }
            frame "Ram Record" {
            }
            frame "HardDisk Record" {
            }
            frame "Disengage Update" {
            }
            frame "Update", Default {
              w363 = u32 2049184 items=["SENSOR MODE"=4212128, "CCD MODE"=4212384, "READOUT MODE"=4211872, "ACTIVE VIEW INDEX"=4343136, "BITS PER CHANNEL"=4342976, "IMAGE PIXEL TYPE"=4343296, "BINNING"=4215968, "EXPOSURE TIME"=2049184, "CONTRAST GAIN"=3163312, "CONTRAST OFFSET"=3163328, "LIGHT MODE"=2114720, "SENSITIVITY"=2114992, "PHOTON IMAGING MODE"=2115200, "HIGH DYNAMIC RANGE MODE"=3163360, "WHITE BALANCE"=3163568, "TEMPERATURE"=2115232, "TEMPERATURE TARGET"=2115264, "SENSOR COOLER FAN"=2115296, "LINEBUNDLE HEIGHT"=4212192, "MECHANICAL SHUTTER"=2115488, "BACK FOCUS POSITION"=8422304, "TRIGGER CONNECTOR"=1066432, "TRIGGER SOURCE"=1066144, "OUTPUT TRIGGER SOURCE"=1852576, "TRIGGER GLOBAL EXPOSURE"=2049680, "FIRST TRIGGER BEHAVIOR"=2049696, "CHANNEL SYNC"=1852352, "READOUT DIRECTION"=4211904, "PRE HSYNC COUNT"=1852704, "INTERNAL LINE SPEED"=4226000, "INTERNAL LINE INTERVAL"=4226016] ("Parameter")
              n70 = Index Array(array=w361) -> (element=w360:T1)  [unwired: 1 in]
              n71 = Unbundle By Name(w360) -> ("Exposure/ms"=w365:dbl)  [unwired: 1 out]
              n72 = Divide(x=w365, y=1000.0) -> (x/y=w362:dbl)
              n73 = call "tm_setparameter_a.vi"("Value in"=w362, "Parameter"=w363, "Handle in"=w367) -> ("Handle out"=w366:u32)  [unwired: 7 in, 1 out]
            }
            frame "ROI" {
            }
            frame "Binning" {
            }
            frame "Scan Mode" {
            }
            frame "Trigger Mode" {
            }
            frame "Readout Mode" {
              w400 = u32 4194832  # Sensor Mode
              w404 = u32 2031888  # Exposure time
              n74 = Index Array(array=w393) -> (element=w392:T1)  [unwired: 1 in]
              n75 = Unbundle By Name(w392) -> ("Exposure/ms"=w413:dbl, "Slit.Slit Width /%"=w409:dbl, "Slit.Scanning Mode"=w398:dbl)
              n76 = call "tm_stopcapture.vi"("error in (no error)"=w414, "Handle in"=w416) -> ("error out"=w417:errorcluster, "Handle out"=w415:u32)  [unwired: 8 in]
              n77 = Divide(x=w413, y=1000.0) -> (x/y=w411:dbl)
              n78 = Multiply(x=w409, y=2048 ("input variable")) -> (x*y=w408:dbl)
              n79 = call "tm_unpreparecapture.vi"("error in (no error)"=w417, "Handle in"=w415) -> ("error out"=w395:errorcluster, "Handle out"=w399:u32)  [unwired: 8 in]
              n80 = call "tm_setpropertyvalue.vi"("error in (no error)"=w395, "Value in"=w398, "Property ID"=w400, "Handle in"=w399) -> ("error out"=w396:errorcluster, "Handle out"=w397:u32)  [unwired: 6 in]
              n81 = Divide(x=w408, y=100.0) -> (x/y=w406:dbl)
              n82 = case shown="12" w398 {
                tunnel: [w422 w423] -> w405
                tunnel: w411 -> [w422 w431]
                tunnel: w406 -> [_ w430]
                tunnel: w397 -> [w421 w425]
                tunnel: [w421 w427] -> w403
                tunnel: [w420 w426] -> w402
                tunnel: w396 -> [w420 w424]
                frame 1, Default {
                }
                frame 12 {
                  w429 = u32 4208720  # Line Interval
                  n83 = formula code="slitExpos=frameInter*LW/(LinesToReadout\n+10+LW);\nlineInter = slitExpos / LW;"("frameInter"=w431, "LW"=w430, "LinesToReadout"=2048 ("input variable")) -> ("slitExpos"=w423:dbl, "lineInter"=w428:dbl)
                  n84 = call "tm_setpropertyvalue.vi"("error in (no error)"=w424, "Value in"=w428, "Property ID"=w429, "Handle in"=w425) -> ("error out"=w426:errorcluster, "Handle out"=w427:u32)  [unwired: 6 in]
                }
              }
              n85 = call "tm_setpropertyvalue.vi"("error in (no error)"=w402, "Value in"=w405, "Property ID"=w404, "Handle in"=w403) -> ("error out"=w401:errorcluster, "Handle out"=w394:u32)  [unwired: 6 in]
            }
            frame "Readout Direction" {
            }
            frame "Preview" {
              n86 = call "tm_waitnextframe.vi"("error in (no error)"=w440, "Timeout"=500, "Handle in"=w446) -> ("error out"=w438:errorcluster, "Handle out"=w445:u32)  [unwired: 5 in, 2 out]
              n87 = case shown="No Error" w438 {
                selector: w438 -> [w449 w463]
                tunnel: w445 -> [w461 w462]
                tunnel: [w460 w462] -> w444
                tunnel: w442 -> [w459 _]
                tunnel: w441 -> [w458 _]
                tunnel: w440 -> [w453 _]
                tunnel: [w450 w463] -> w439
                frame No Error {
                  w455 = 0 ("Timeout")
                  n88 = call "tm_getframe_a.vi"("error in (no error)"=w449, "Buffer Info"=w459, "Handle in"=w461) -> ("error out"=w451:errorcluster, "Data 16"=w456:u16[][], "Handle out"=w460:u32)  [unwired: 4 in, 2 out]
                  n89 = Bundle("State"=Stack_Track."Display", "Timeout"=w455, "Data 16"=w456, "Timeout"=w455) -> (w454:T16)  [unwired: 1 in]
                  n90 = Enqueue Element(queue=w458, element=w454, error in (no error)=w453) -> (error out=w452:errorcluster)  [unwired: 1 in, 2 out]
                  n91 = Merge Errors(w451, w452) -> (w450:errorcluster)
                }
                frame Error {
                }
              }
            }
            frame "ROIWindow" {
            }
            frame "Trigger Source" {
              (unwired) u32 1066144 items=["SENSOR MODE"=4212128, "CCD MODE"=4212384, "READOUT MODE"=4211872, "ACTIVE VIEW INDEX"=4343136, "BITS PER CHANNEL"=4342976, "IMAGE PIXEL TYPE"=4343296, "BINNING"=4215968, "EXPOSURE TIME"=2049184, "CONTRAST GAIN"=3163312, "CONTRAST OFFSET"=3163328, "LIGHT MODE"=2114720, "SENSITIVITY"=2114992, "PHOTON IMAGING MODE"=2115200, "HIGH DYNAMIC RANGE MODE"=3163360, "WHITE BALANCE"=3163568, "TEMPERATURE"=2115232, "TEMPERATURE TARGET"=2115264, "SENSOR COOLER FAN"=2115296, "LINEBUNDLE HEIGHT"=4212192, "MECHANICAL SHUTTER"=2115488, "BACK FOCUS POSITION"=8422304, "TRIGGER CONNECTOR"=1066432, "TRIGGER SOURCE"=1066144, "OUTPUT TRIGGER SOURCE"=1852576, "TRIGGER GLOBAL EXPOSURE"=2049680, "FIRST TRIGGER BEHAVIOR"=2049696, "CHANNEL SYNC"=1852352, "READOUT DIRECTION"=4211904, "PRE HSYNC COUNT"=1852704, "INTERNAL LINE SPEED"=4226000, "INTERNAL LINE INTERVAL"=4226016] ("Parameter")
              w478 = 1 items=["Snap", "Sequence"] ("Capture mode")
              n92 = Index Array(array=w470) -> (element=w469:T1)  [unwired: 1 in]
              n93 = Unbundle By Name(w469) -> ("Mode"=w472:enum16{"X", "XY", "XYZ", "XYZT", "XYZC"})
              n94 = call "tm_stopcapture.vi"("error in (no error)"=w479, "Handle in"=w482) -> ("error out"=w486:errorcluster, "Handle out"=w487:u32)  [unwired: 8 in]
              n95 = call "tm_unpreparecapture.vi"("error in (no error)"=w486, "Handle in"=w487) -> ("error out"=w474:errorcluster, "Handle out"=w477:u32)  [unwired: 8 in]
              n96 = case shown="\"XYZT\"" w472 {
                tunnel: [T9 {"Mode"=2, "Polarity"=2, "Times"=2, "Delay"=0.0} ("Parameters") T9 {"Mode"=2, "Polarity"=2, "Times"=2, "Delay"=0.0} ("Parameters") T9 {"Mode"=2, "Polarity"=2, "Times"=2, "Delay"=0.0} ("Parameters") T9 {"Mode"=1, "Polarity"=2, "Times"=2, "Delay"=0.0} ("Parameters") T9 {"Mode"=1, "Polarity"=2, "Times"=2, "Delay"=0.0} ("Parameters")] -> w475
                tunnel: [CameraControlTypeDef."Preview" ("Enum") CameraControlTypeDef."Idle" ("Enum") CameraControlTypeDef."Idle" ("Enum") CameraControlTypeDef."Idle" ("Enum") CameraControlTypeDef."Preview" ("Enum")] -> w471
                frame "XY", Default {
                }
                frame "XYZT" {
                }
                frame "XYZ" {
                }
                frame "XYZC" {
                }
                frame "X" {
                }
              }
              n97 = call <userlib>:"tm_setinputtrigger.vi"("error in (no error)"=w474, "Parameters"=w475, "Handle in"=w477) -> ("error out"=w473:errorcluster, "Handle out"=w476:u32)  [unwired: 7 in]
              n98 = call "tm_preparecapture.vi"("error in (no error)"=w473, "Capture mode"=w478, "Handle in"=w476) -> ("error out"=w485:errorcluster, "Buffer Info"=w483:T5, "Handle out"=w484:u32)  [unwired: 5 in, 1 out]
              n99 = call "tm_startcapture_b.vi"("error in (no error)"=w485, "Handle in"=w484) -> ("error out"=w480:errorcluster, "Handle out"=w481:u32)  [unwired: 8 in]
            }
          }
          n100 = local read "stop"() -> (w313:bool)
        }
        n101 = while {
          tunnel: w140 -> [w181]
          shift-right: [w178] -> _
          shift-left: _ -> [w177]
          tunnel: w147 -> [w176]
          shift-right: [w172] -> w141
          shift-left: w144 -> [w171]
          shift-right: [w175] -> _
          shift-left: w146 -> [w174]
          shift-right: [w170] -> w142
          shift-left: w143 -> [w169]
          tunnel: [w168] -> w139
          shift-right: [w167] -> w138
          shift-left: _ -> [w166]
          stop <- w165 stop-if-true
          n102 = Dequeue Element(queue=w181, timeout in ms (-1)=1) -> (queue out=w168:refnum<queue>, element=w180:T15)  [unwired: 1 in, 2 out]
          n103 = Unbundle(w180) -> ("Mode"=w179:T7, "Microscope Settings Array"=w164:T1[])
          n104 = case shown="\"generateWaves\"" w179 {
            tunnel: [_ _ _ TRUE] -> _
            tunnel: w164 -> [_ w188 w237 _]
            tunnel: [w186 w200 w266 w287] -> w178
            tunnel: w177 -> [w186 w192 w266 w287]
            tunnel: w176 -> [_ _ _ _]
            tunnel: w168 -> [_ w191 w267 _]
            tunnel: [w183 w196 w246 w286] -> w170
            tunnel: [w184 w194 w261 w285] -> w172
            tunnel: w171 -> [w184 w193 w268 w285]
            tunnel: [w185 w199 w248 w284] -> w175
            tunnel: w174 -> [w185 w198 w248 w284]
            tunnel: w169 -> [w183 w197 w257 w286]
            tunnel: [w182 w190 w243 w282] -> w167
            tunnel: w166 -> [w182 w190 w242 w282]
            frame "Idle", Default {
            }
            frame "generateWaves" {
              n105 = Index Array(array=w188) -> (element=w187:T1)  [unwired: 1 in]
              n106 = Unbundle By Name(w187) -> ("Mode"=w195:enum16{"X", "XY", "XYZ", "XYZT", "XYZC"})
              n107 = case shown="\"XY\", Default" w195 {
                tunnel: [w205 w226] -> w200
                tunnel: w187 -> [_ w206]
                tunnel: [w203 w217] -> w199
                tunnel: w198 -> [w203 _]
                tunnel: w197 -> [w204 w232]
                tunnel: [w204 w232] -> w196
                tunnel: [w201 w231] -> w194
                tunnel: w193 -> [w202 w231]
                tunnel: w192 -> [w205 _]
                tunnel: w191 -> [_ _]
                tunnel: [_ w212] -> w189
                frame "X" {
                  n108 = call "Calibration.vi"("Analogue In"=w202) -> ("Analogue In Out"=w201:refnum<k21>)
                }
                frame "XY", Default {
                  w214 = 10.0  # Piezo Factor
                  # "XY Mirrors"
                  n109 = Unbundle By Name(w206) -> ("Piezo Position /um"=w207:dbl, "Exposure/ms"=w209:dbl, "Samples per millisecond"=w208:dbl, "Camera Delay"=w210:dbl, "Relax/ms"=w211:dbl)
                  n110 = Divide(x=w207, y=w214) -> (x/y=w213:dbl)
                  n111 = call "XY Galvo With Homography.vi"("Exposure (ms)"=w209, "Camera Delay /ms"=w210, "Samples /Millisecond"=w208, "Relax (ms)"=w211, "Piezo Position (um)"=w213) -> ("Scan Mirror Signal"=w236:dbl[], "Piezo Signal"=w230:dbl[], "Camera Signal"=w219:dbl[], "Laser Signal"=w224:dbl[], "Z Mirror Signal"=w235:dbl[])  [unwired: 10 in]
                  n112 = Divide(x=0.001 ("y"), y=w208) -> (x/y=w218:dbl)
                  n113 = Bundle By Name("Y"=w236, "dt"=w218) -> (w233:waveform(dbl))  [unwired: 1 in]
                  n114 = Bundle By Name("Y"=w230, "dt"=w218) -> (w229:waveform(dbl))  [unwired: 1 in]
                  n115 = Bundle By Name("Y"=w235, "dt"=w218) -> (w234:waveform(dbl))  [unwired: 1 in]
                  n116 = Build Array(w219) -> (w220:dbl[][])
                  n117 = Build Array(w224) -> (w227:dbl[][])
                  n118 = Transpose 2D Array(2D array=w220) -> (transposed array=w222:dbl[][])
                  n119 = Transpose 2D Array(2D array=w227) -> (transposed array=w223:dbl[][])
                  n120 = Bundle By Name("data"=w222) -> (w221:digitaldata)  [unwired: 1 in]
                  n121 = Bundle By Name("data"=w223) -> (w225:digitaldata)  [unwired: 1 in]
                  n122 = Bundle By Name("Y"=w221, "dt"=w218) -> (w216:digitalwaveform)  [unwired: 1 in]
                  n123 = Bundle By Name("Y"=w225, "dt"=w218) -> (w215:digitalwaveform)  [unwired: 1 in]
                  n124 = Build Array(w233, w234, w229) -> (w226:waveform(dbl)[])
                  n125 = Build Array(w216, w215) -> (w217:digitalwaveform[])
                  n126 = Bundle(w226, "Digital Waveform"=w216, "Digital Waveform"=w215) -> (w212:T17)  [unwired: 1 in]
                }
              }
              n127 = call "Graph.vi"("Cluster"=w189) -> ()
            }
            frame "runWaves" {
              n128 = Index Array(array=w237) -> (element=w238:T1)  [unwired: 1 in]
              n129 = Unbundle By Name(w238) -> ("Samples per millisecond"=w239:dbl)
              n130 = Index Array(array=w266, index=0) -> (element=w264:waveform(dbl))
              n131 = Multiply(x=w239, y=1000.0) -> (x*y=w259:dbl)
              n132 = local read "Scan Continuously"() -> (w260:bool)
              n133 = call-poly <vilib>:"Number of Waveform Samples.vi"("waveform in"=w264) -> ("number of samples"=w240:i32)  [unwired: 8 in, 2 out]
              n134 = call-poly <vilib>:"DAQmx Timing.vi"("task/channels in"=w268, "samples per channel"=w240, "rate"=w259, "error in"=w242) -> ("task out"=w271:refnum<k21>, "error out"=w263:errorcluster)  [unwired: 10 in]
              n135 = call-poly <vilib>:"DAQmx Timing.vi"("task/channels in"=w257, "samples per channel"=w240, "rate"=w259, "error in"=w242) -> ("task out"=w258:refnum<k21>, "error out"=w255:errorcluster)  [unwired: 10 in]
              n136 = case shown="True" w260 {
                tunnel: w267 -> [w273 w281]
                tunnel: [w274 w280] -> _
                tunnel: w237 -> [w275 w279]
                frame False {
                  n137 = Bundle("Mode"=ModeEnum."Idle", "Microscope Settings Array"=w275) -> (w276:T15)  [unwired: 1 in]
                  n138 = Enqueue Element(queue=w273, element=w276) -> (queue out=w274:refnum<queue>)  [unwired: 2 in, 2 out]
                }
                frame True {
                  n139 = Bundle("Mode"=ModeEnum."runWaves", "Microscope Settings Array"=w279) -> (w278:T15)  [unwired: 1 in]
                  n140 = Enqueue Element(queue=w281, element=w278) -> (queue out=w280:refnum<queue>)  [unwired: 2 in, 2 out]
                }
              }
              n141 = call-poly <vilib>:"DAQmx Write.vi"("task/channels in"=w271, "data"=w266, "error in"=w263) -> ("task out"=w250:refnum<k21>, "error out"=w253:errorcluster)  [unwired: 10 in, 1 out]
              n142 = call-poly <vilib>:"DAQmx Write.vi"("task/channels in"=w258, "data"=w248, "error in"=w255) -> ("task out"=w249:refnum<k21>, "error out"=w252:errorcluster)  [unwired: 10 in, 1 out]
              n143 = Merge Errors(w253, w252) -> (w251:errorcluster)
              n144 = call <vilib>:"DAQmx Start Task.vi"("task/channels in"=w250, "error in"=w251) -> ("task out"=w270:refnum<k21>, "error out"=w269:errorcluster)  [unwired: 12 in]
              n145 = call <vilib>:"DAQmx Start Task.vi"("task/channels in"=w249, "error in"=w251) -> ("task out"=w256:refnum<k21>, "error out"=w254:errorcluster)  [unwired: 12 in]
              n146 = call <vilib>:"DAQmx Wait Until Done.vi"("task/channels in"=w270, "error in"=w269) -> ("task out"=w262:refnum<k21>, "error out"=w245:errorcluster)  [unwired: 12 in]
              n147 = call <vilib>:"DAQmx Wait Until Done.vi"("task/channels in"=w256, "error in"=w254) -> ("task out"=w247:refnum<k21>, "error out"=w244:errorcluster)  [unwired: 12 in]
              n148 = call <vilib>:"DAQmx Stop Task.vi"("task/channels in"=w262) -> ("task out"=w261:refnum<k21>)  [unwired: 13 in, 1 out]
              n149 = Merge Errors(w245, w244) -> (w243:errorcluster)
              n150 = call <vilib>:"DAQmx Stop Task.vi"("task/channels in"=w247) -> ("task out"=w246:refnum<k21>)  [unwired: 13 in, 1 out]
            }
            frame "stop" {
            }
          }
          n151 = local read "stop"() -> (w165:bool)
        }
        n152 = while "Tiff Consumer" {
          tunnel: [w291] -> w160
          tunnel: [w294] -> w157
          tunnel: w150 -> [w296]
          tunnel: w149 -> [w288]
          stop <- w298 stop-if-true
          # "Delay, maybe?\nCheck"
          n153 = Dequeue Element(queue=w296, timeout in ms (-1)=1) -> (queue out=w293:refnum<queue>, element=w295:T10, error out=w292:errorcluster)  [unwired: 1 in, 1 out]
          n154 = Unbundle By Name(w295) -> ("State"=w289:T11, "Image"=w290:u16[][])  [unwired: 1 out]
          n155 = case shown="\"Idle\", Default" w289 {
            selector: w289 -> [_ w309 w310]
            tunnel: [w306 w308 w311] -> w294
            tunnel: w293 -> [w306 w308 w311]
            tunnel: [Stack_Track."Idle" ("State") w309 w310] -> _
            tunnel: w290 -> [w301 _ _]
            tunnel: w288 -> [w305 _ _]
            tunnel: w292 -> [w304 w307 w312]
            tunnel: [w303 w307 w312] -> w291
            frame "Display" {
              n156 = call "IMAQ ArrayToImage"("Image Pixels (U16)"=w301, "error in (no error)"=w304, "Image"=w305) -> ("error out"=w303:errorcluster, "Image Out"=w300:T3)  [unwired: 7 in]
              "Image" <- w300
              n157 = call "IMAQ Histograph"("Image"=w300) -> ("Histogram Graph"=→"Histogram":T4)  [unwired: 7 in, 3 out]
            }
            frame "Idle", Default {
            }
            frame "Start Sequence" {
            }
          }
          n158 = local read "stop"() -> (w298:bool)
        }
        n159 = Merge Errors(w159, w160, w138) -> (w161:errorcluster)
      }
      frame "deinit" {
        n160 = call <vilib>:"DAQmx Stop Task.vi"("task/channels in"=w547) -> ("task out"=w548:refnum<k21>)  [unwired: 13 in, 1 out]
        n161 = call <vilib>:"DAQmx Stop Task.vi"("task/channels in"=w549) -> ("task out"=w550:refnum<k21>)  [unwired: 13 in, 1 out]
        n162 = call <vilib>:"DAQmx Clear Task.vi"("task in"=w548) -> ("error out"=w544:errorcluster)  [unwired: 14 in]
        n163 = call "tm_stopcapture.vi"("error in (no error)"=w559, "Handle in"=w555) -> ("error out"=w562:errorcluster, "Handle out"=w561:u32)  [unwired: 8 in]
        n164 = call <vilib>:"DAQmx Clear Task.vi"("task in"=w550) -> ("error out"=w545:errorcluster)  [unwired: 14 in]
        n165 = call "tm_unpreparecapture.vi"("error in (no error)"=w562, "Handle in"=w561) -> ("error out"=w563:errorcluster, "Handle out"=w560:u32)  [unwired: 8 in]
        n166 = call "tm_closecamera.vi"("error in (no error)"=w563, "Handle in"=w560) -> ("error out"=w564:errorcluster)  [unwired: 9 in]
        n167 = Flush Queue(queue=w537) -> (queue out=w543:refnum<queue>)  [unwired: 1 in, 2 out]
        n168 = call "tm_deinitialize.vi"("error in (no error)"=w564) -> ("error out"=w540:errorcluster)  [unwired: 10 in]
        n169 = Release Queue(queue=w538, error in (no error)=w540) -> (error out=w557:errorcluster)  [unwired: 1 in, 2 out]
        n170 = Release Queue(queue=w543) -> (error out=w546:errorcluster)  [unwired: 2 in, 2 out]
        n171 = Flush Queue(queue=w542, error in (no error)=w540) -> (queue out=w541:refnum<queue>, error out=w539:errorcluster)  [unwired: 1 out]
        n172 = Release Queue(queue=w541, error in (no error)=w539) -> (error out=w556:errorcluster)  [unwired: 1 in, 2 out]
        n173 = Merge Errors(w557, w556, w546, w545, w544) -> (w558:errorcluster)
      }
    }
    n174 = Or(x="stop", y=w17) -> (x .or. y?=w18:bool)
  }
  "error IO" <- w5
  n175 = disable-structure shown="Enabled" {
    frame Disabled {
      # "Parallise decode buffer"
      n176 = call "tm_startcapture_b.vi"() -> ()  [unwired: 10 in, 2 out]
      n177 = call "tm_waitnextframe.vi"() -> ()  [unwired: 8 in, 4 out]
      n178 = call "tm_getframe_a.vi"() -> ()  [unwired: 7 in, 5 out]
    }
    frame Enabled {
    }
  }
  n179 = property on="stop" class="Bool (strict)" props=["Value"]() -> ()  [unwired: 2 in, 3 out]
